vi "SSH_TUNNEL_Connect.vi"(8 "error in (no error)":errorcluster, 9 "MIDAS Port Number":u16, 10 "MIDAS Address":string, 11 "SSH_TUNNEL in":refnum<class "SSH_TUNNEL.lvclass">) -> (0 "error out":errorcluster, 2 "MIDAS Address":string, 3 "SSH_TUNNEL out":refnum<class "SSH_TUNNEL.lvclass">)   [LabVIEW 2018, in "SSH_TUNNEL.lvclass"]
uses:
  SSH_TUNNEL.lvclass
  SSH_TUNNEL.lvclass/SSH_TUNNEL.ctl
panel:
  out "standard error 2":string
  out "standard output 2":string
  out "standard output":string
  out "plink command (passwd hashed out)":string
  out "standard error":string
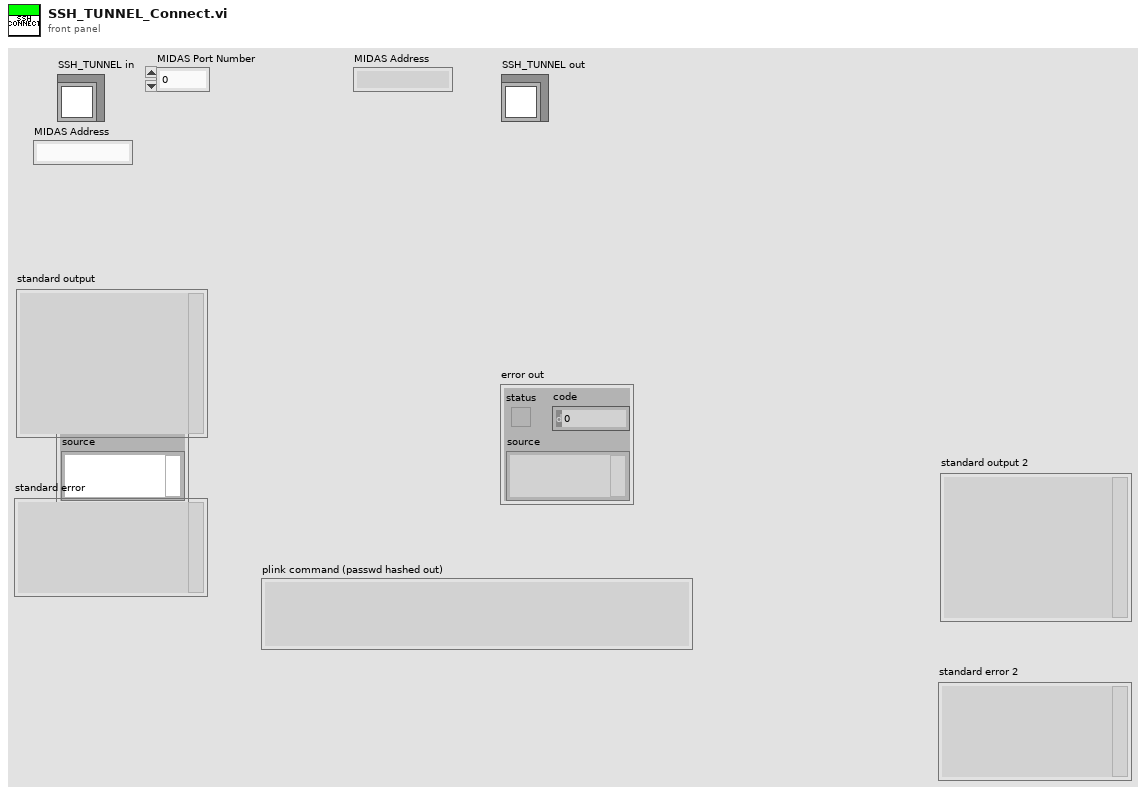
[diagram p1: front panel]
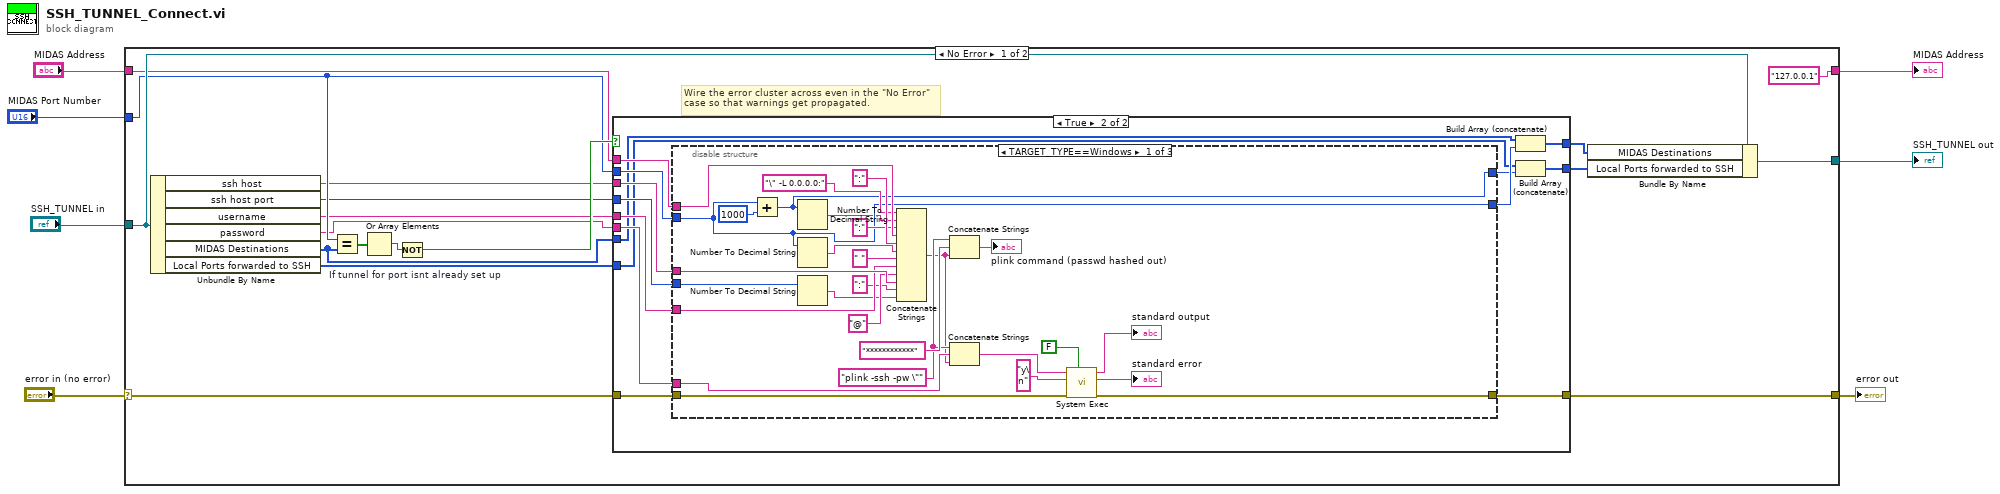
[diagram p0: block diagram]
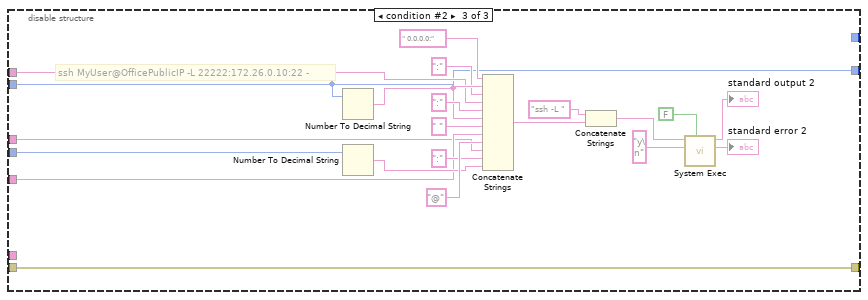
[diagram p4: hidden frame]
diagram:
  n1 = case shown="No Error" "error in (no error)" {
    selector: "error in (no error)" -> [w9 w95]
    tunnel: [w8 w95] -> w6
    tunnel: [w22 w94] -> w4
    tunnel: "SSH_TUNNEL in" -> [w23 w94]
    tunnel: "MIDAS Address" -> [w17 w93]
    tunnel: ["127.0.0.1" ("MIDAS Address 2") w93] -> w2
    tunnel: "MIDAS Port Number" -> [w18 _]
    frame No Error {
      # "Wire the error cluster across even in the \"No Error\"\ncase so that warnings get propagated."
      n2 = Unbundle By Name(w23) -> ("ssh host"=w14:string, "ssh host port"=w13:i32, "username"=w15:string, "password"=w16:string, "MIDAS Destinations"=w24:u16[], "Local Ports forwarded to SSH"=w11:u16[])
      n3 = Equal?(x=w18, y=w24) -> (x = y?=w19:bool[])
      n4 = Or Array Elements(Boolean array=w19) -> (logical OR=w20:bool)
      n5 = Not "If tunnel for port isnt already set up"(x=w20) -> (.not. x?=w21:bool)
      n6 = case shown="True" w21 {
        tunnel: w18 -> [_ w42]
        tunnel: w17 -> [_ w41]
        tunnel: w16 -> [_ w40]
        tunnel: w15 -> [_ w39]
        tunnel: w14 -> [_ w38]
        tunnel: w13 -> [_ w37]
        tunnel: w24 -> [w28 w36]
        tunnel: [w28 w34] -> w12
        tunnel: w11 -> [w27 w33]
        tunnel: [w27 w31] -> w10
        tunnel: w9 -> [w26 w30]
        tunnel: [w26 w29] -> w8
        frame False {
        }
        frame True {
          n7 = disable-structure shown="TARGET_TYPE==Windows" {
            disable-tunnel: w40 -> [w54 _ _]
            disable-tunnel: w39 -> [w68 _ w78]
            disable-tunnel: w38 -> [w70 _ w77]
            disable-tunnel: w42 -> [w48 _ w75]
            disable-tunnel: w41 -> [w65 _ w79]
            disable-tunnel: w37 -> [w56 _ w76]
            disable-tunnel: [w48 _ w75] -> w35
            disable-tunnel: [w45 _ _] -> w32
            disable-tunnel: w30 -> [w44 w71 w72]
            disable-tunnel: [w43 w71 w72] -> w29
            frame condition #0 (active) {
              w51 = "plink -ssh -pw \"" ("string")
              n8 = Add(x=w48, y=u16 1000) -> (x+y=w45:u16)
              n9 = Number To Decimal String(number=w45) -> (decimal integer string=w46:string)  [unwired: 1 in]
              n10 = Number To Decimal String(number=w48) -> (decimal integer string=w58:string)  [unwired: 1 in]
              n11 = Number To Decimal String(number=w56) -> (decimal integer string=w62:string)  [unwired: 1 in]
              n12 = Concatenate Strings("\" -L 0.0.0.0:" ("string"), w46, ":" ("string"), w65, ":" ("string"), w58, " " ("string"), w68, "@" ("string"), w70, ":" ("string"), w62) -> (w50:string)
              n13 = Concatenate Strings(w51, "************" ("string"), w50) -> (→"plink command (passwd hashed out)":string)
              n14 = Concatenate Strings(w51, w54, w50) -> (w49:string)
              n15 = call <vilib>:"System Exec.vi"("wait until completion? (T)"=FALSE, "error in (no error)"=w44, "standard input"="y\n", "command line"=w49) -> ("error out"=w43:errorcluster, "standard error"=→"standard error":string, "standard output"=→"standard output":string)  [unwired: 4 in, 1 out]
            }
            frame condition #1 {
            }
            frame condition #2 {
              # "ssh MyUser@OfficePublicIP -L 22222:172.26.0.10:22 -"
              n16 = Number To Decimal String(number=w75) -> (decimal integer string=w83:string)  [unwired: 1 in]
              n17 = Number To Decimal String(number=w76) -> (decimal integer string=w87:string)  [unwired: 1 in]
              n18 = Concatenate Strings(" 0.0.0.0:" ("string"), w83, ":" ("string"), w79, ":" ("string"), w83, " " ("string"), w78, "@" ("string"), w77, ":" ("string"), w87) -> (w74:string)
              n19 = Concatenate Strings("ssh -L " ("string"), w74) -> (w73:string)
              n20 = call <vilib>:"System Exec.vi"("wait until completion? (T)"=FALSE, "standard input"="y\n", "command line"=w73) -> ("standard error"=→"standard error 2":string, "standard output"=→"standard output 2":string)  [unwired: 5 in, 2 out]
            }
          }
          n21 = Build Array (concatenate)(w36, w35) -> (w34:u16[])
          n22 = Build Array (concatenate)(w33, w32) -> (w31:u16[])
        }
      }
      n23 = Bundle By Name(cluster=w23, "MIDAS Destinations"=w12, "Local Ports forwarded to SSH"=w10) -> (w22:refnum<class "SSH_TUNNEL.lvclass">)
    }
    frame Error {
    }
  }
  "error out" <- w6
  "SSH_TUNNEL out" <- w4
  "MIDAS Address" <- w2
